vi "Temp.vi"() -> ()   [LabVIEW 2012, in "Galvo.lvclass"]
uses:
  Galvo.lvclass
  <vilib>/DAQmx/configure/timing.llb/DAQmx Timing (Sample Clock).vi
  <vilib>/DAQmx/create/channels.llb/DAQmx Create Channel (DI-Digital Input).vi
  <vilib>/DAQmx/configure/trigger.llb/DAQmx Start Trigger (Digital Edge).vi
panel:
  in  "DAQ cluster":T1={"Physical channels"="", "Custom scale name"="", "Units"=10348, "Minimum value"=0.0, "Maximum value"=0.0, "Timing cluster"={"Sampling rate"=1000.0, "Clock source"="", "Samples per channel"=1000, "Sample mode"=10178}, "Trigger cluster"={"Source"="", "Edge"=10280}} {"Trigger cluster"."Edge" items=["Rising"=10280, "Falling"=10171]; "Timing cluster"."Sample mode" items=["Finite Samples"=10178, "Continuous Samples"=10123, "Hardware Timed Single Point"=12522]; "Timing cluster"."Sampling rate" format="%0.2f"; "Units" items=["Volts"=10348, "From Custom Scale"=10065]}
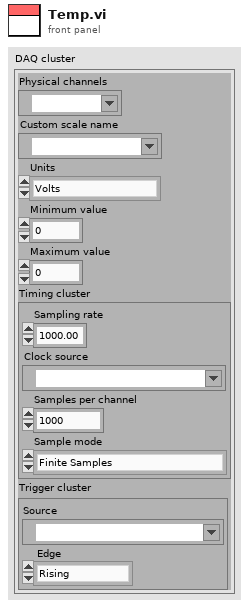
[diagram p1: front panel]
types:
  T1 = cluster{"Physical channels":tag, "Custom scale name":tag, "Units":i32, "Minimum value":dbl, "Maximum value":dbl, "Timing cluster":cluster{"Sampling rate":dbl, "Clock source":tag, "Samples per channel":i32, "Sample mode":i32}, "Trigger cluster":cluster{"Source":tag, "Edge":i32}}
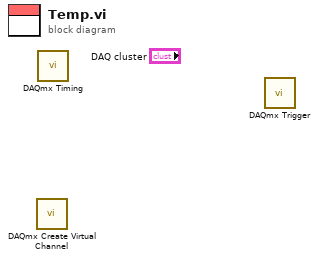
[diagram p0: block diagram]
diagram:
  n1 = call-poly <vilib>:"DAQmx Create Virtual Channel.vi"() -> ()  [unwired: 14 in, 2 out]
  n2 = call-poly <vilib>:"DAQmx Timing.vi"() -> ()  [unwired: 14 in, 2 out]
  n3 = call-poly <vilib>:"DAQmx Trigger.vi"() -> ()  [unwired: 14 in, 2 out]
